vi "Assemble.vi"() -> ()   [LabVIEW 2010]
uses:
  <vilib>/Utility/VariantDataType/VariantType.lvlib
panel:
  out "Result: XML Footer":string
  out "Result: XML Header":string
  out "XML-String-out":string
  out "output array":variant[](array[variant])
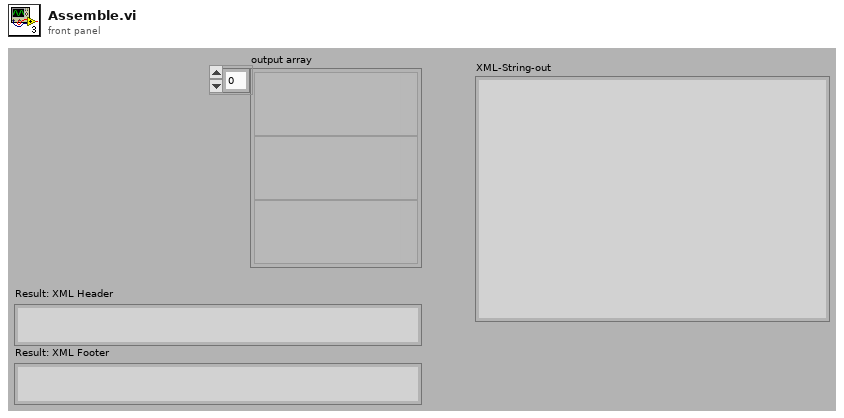
[diagram p1: front panel]
types:
  T1 = cluster{"parameter":string, "type info":string}[]
  T2 = typedef "VariantType.lvlib/Type.ctl" = enum8{"Invalid Type", "Void", "I8", "I16", "I32", "I64", "U8", "U16", "U32", "U64", "Single Float", "Double Float", "Extended Float", "Single Complex", "Double Complex", "Extended Complex", "Enum U8", "Enum U16", "Enum U32", "Enum U64", "Single Float With Unit", "Double Float With Unit", "Extended Float With Unit", "Single Complex with Unit", "Double Complex with Unit", "Extended Complex with Unit", "Boolean", "String", "Path", "Picture", "Tag", "Array", "Cluster", "Variant", "LV Variant", "Waveform", "Timestamp", "Digital Waveform", "Digital Data", "ExpressData", "Refnum", "External Data", "VI", "Poly VI", "LabVIEW Class Instance", "Fixed Point"}
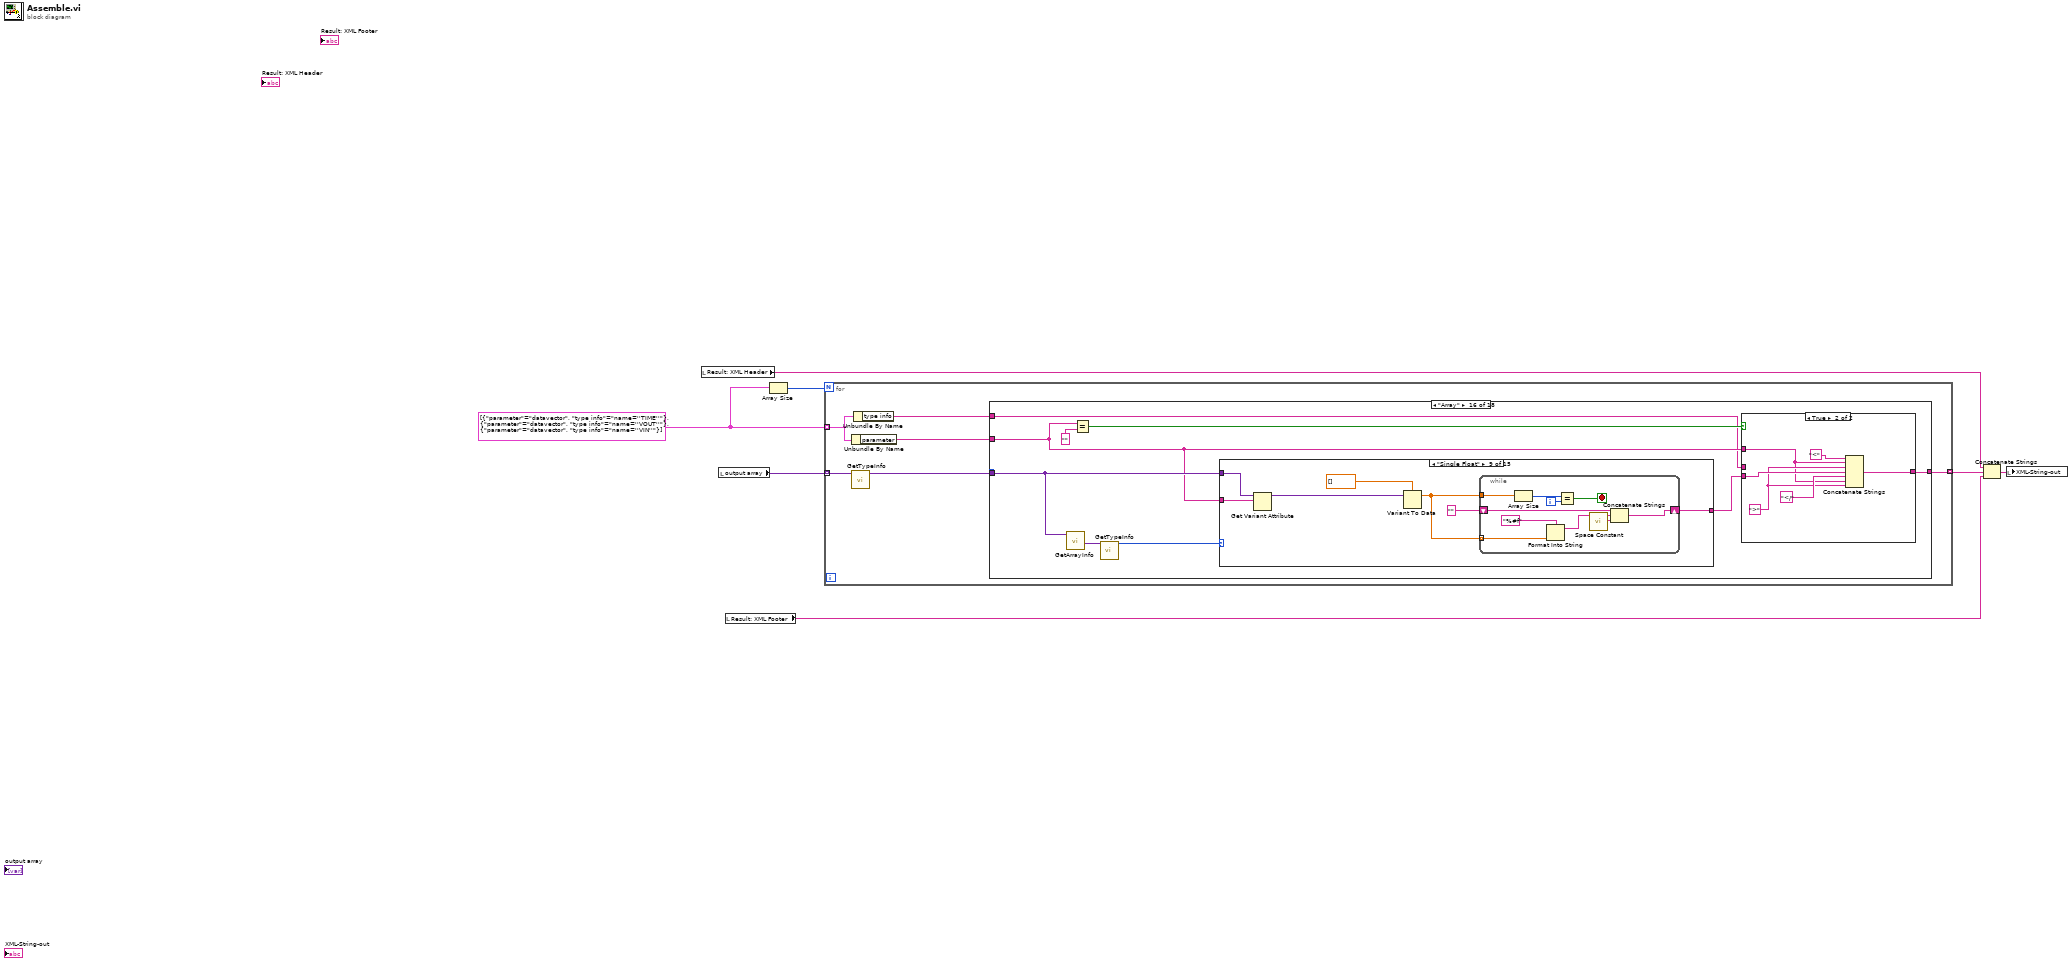
[diagram p0: block diagram]
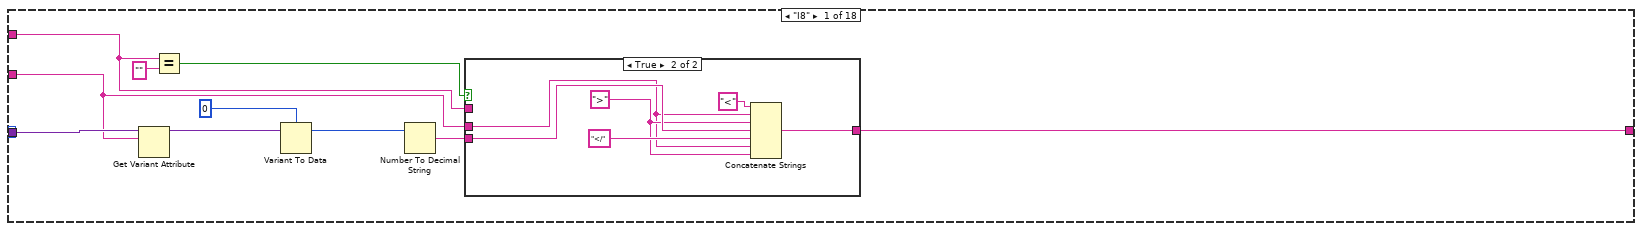
[diagram p2: hidden frame]
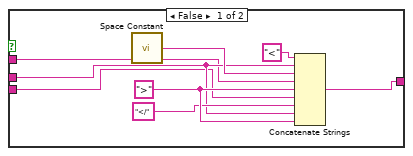
[diagram p3: hidden frame]
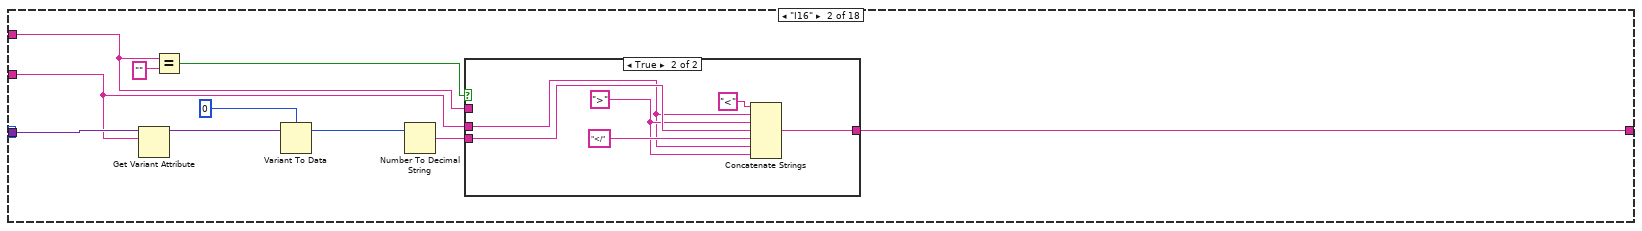
[diagram p4: hidden frame]
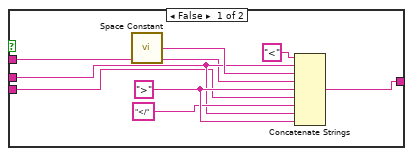
[diagram p5: hidden frame]
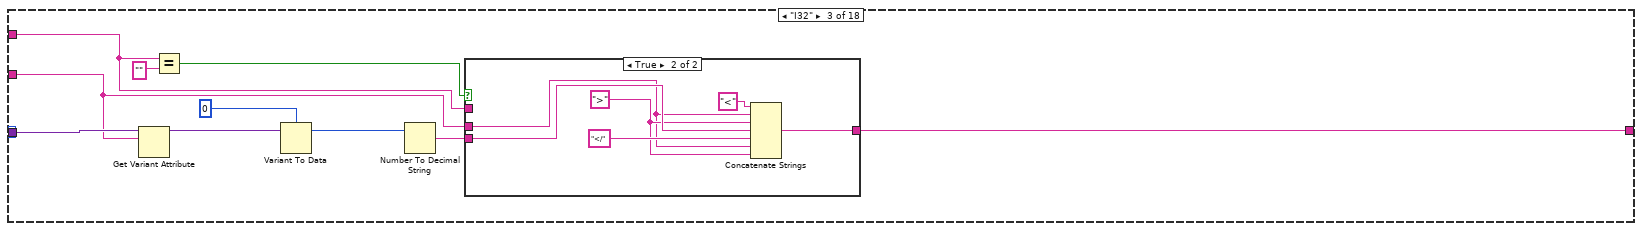
[diagram p6: hidden frame]
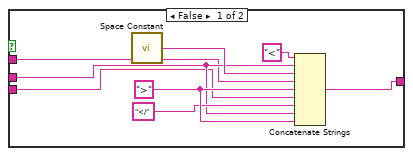
[diagram p7: hidden frame]
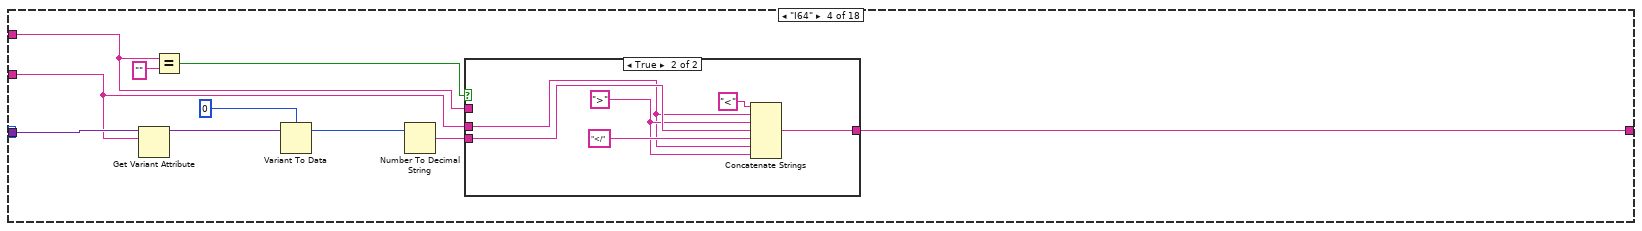
[diagram p8: hidden frame]
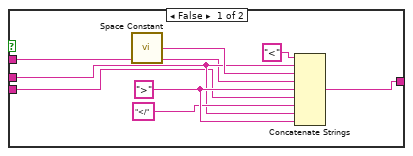
[diagram p9: hidden frame]
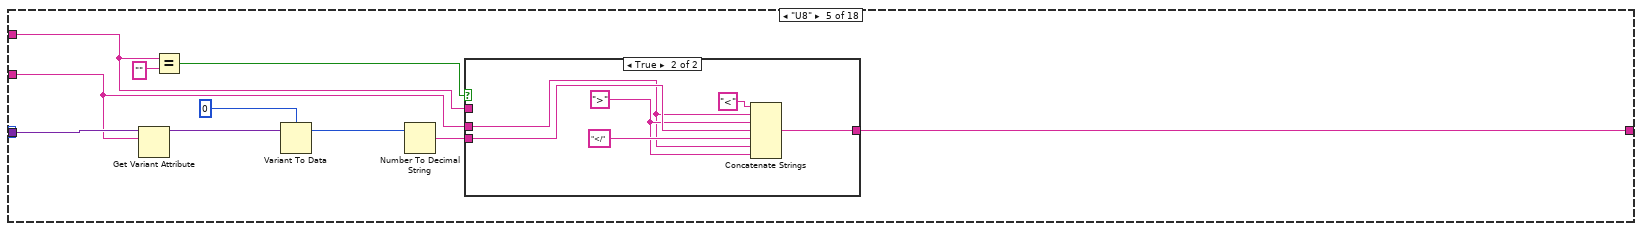
[diagram p10: hidden frame]
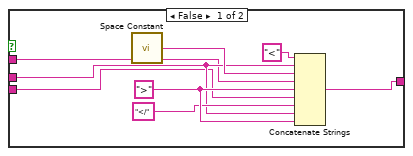
[diagram p11: hidden frame]
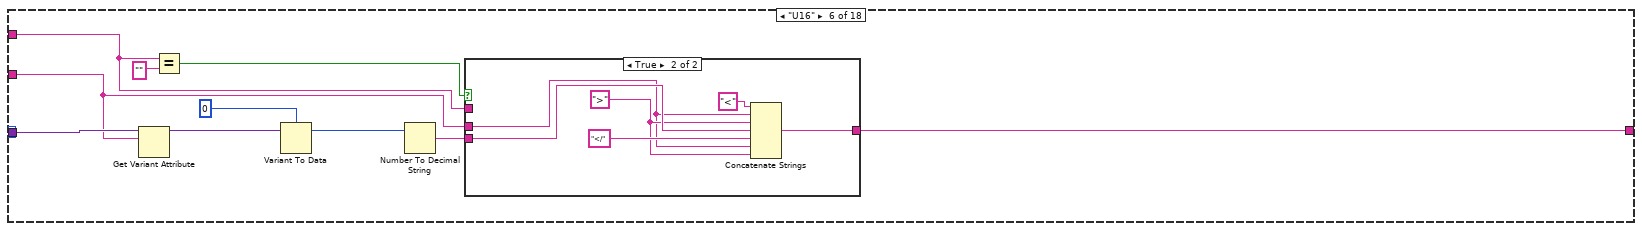
[diagram p12: hidden frame]
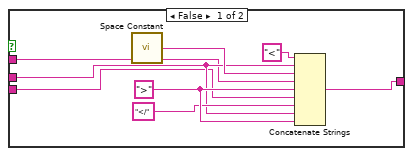
[diagram p13: hidden frame]
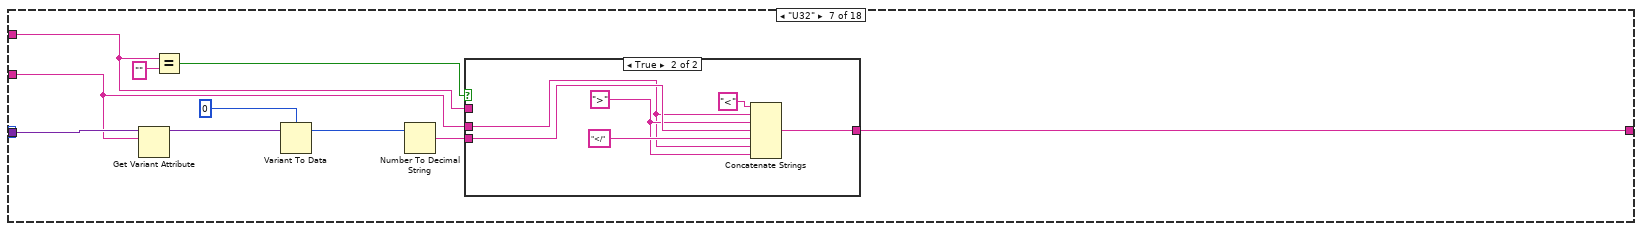
[diagram p14: hidden frame]
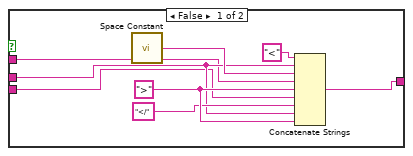
[diagram p15: hidden frame]
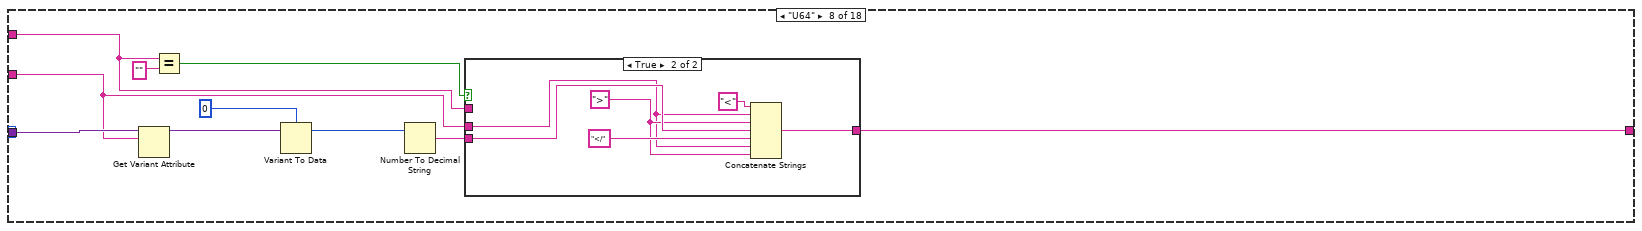
[diagram p16: hidden frame]
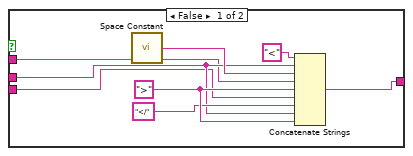
[diagram p17: hidden frame]
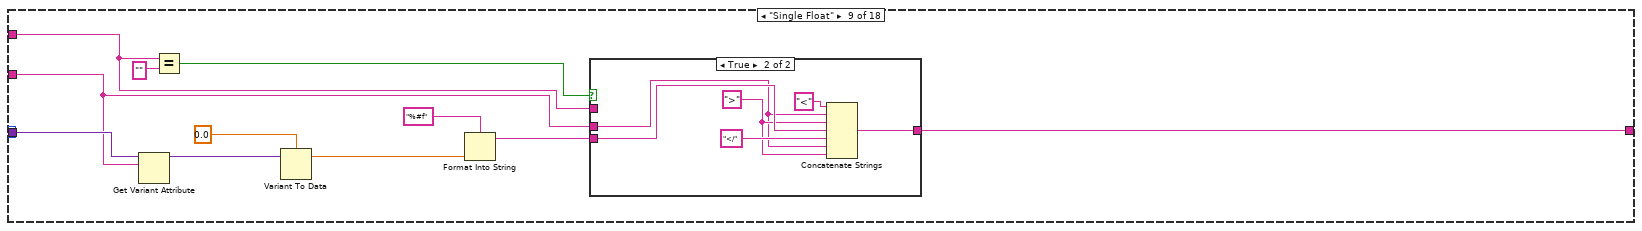
[diagram p18: hidden frame]
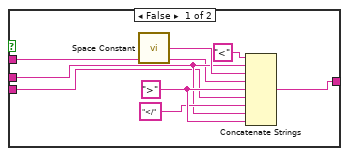
[diagram p19: hidden frame]
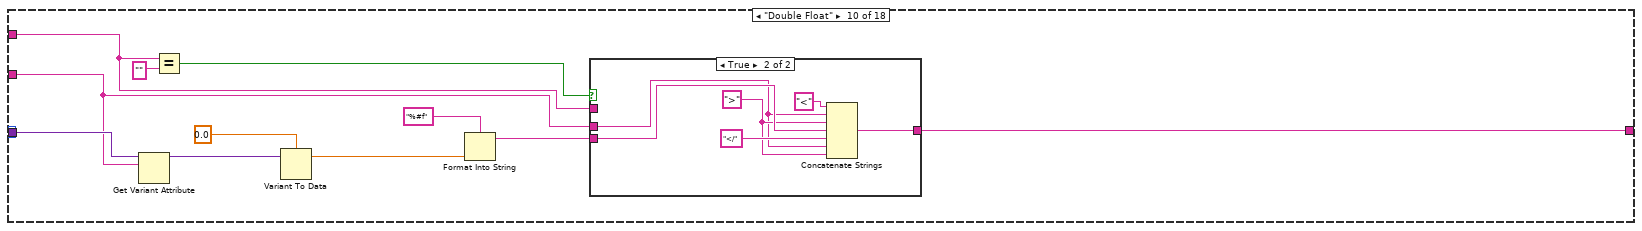
[diagram p20: hidden frame]
diagram:
  w1 = T1 [{"parameter"="datavector", "type info"="name=''TIME''"}, {"parameter"="datavector", "type info"="name=''VOUT''"}, {"parameter"="datavector", "type info"="name=''VIN''"}] ("Parameter out 2")
  n1 = local read "Result: XML Header"() -> (w3:string)
  n2 = local read "output array"() -> (w4:variant[])
  n3 = local read "Result: XML Footer"() -> (w2:string)
  n4 = Array Size(array=w1) -> (size(s)=w7:i32)
  n5 = for {
    N: w7 -> [_]
    tunnel: w4 -> [w11] mode=indexing
    tunnel: w1 -> [w9] mode=indexing
    tunnel: [w13] -> w5 mode=indexing
    n6 = Unbundle By Name(w9) -> ("parameter"=w12:string)
    n7 = call <vilib>:"GetTypeInfo.vi"("Variant"=w11) -> ("Type Enum"=w10:T2)  [unwired: 6 in, 4 out]
    n8 = Unbundle By Name(w9) -> ("type info"=w8:string)
    n9 = case shown="\"Array\"" w10 {
      tunnel: w12 -> [w15 w39 w64 w87 w112 w135 w159 w183 w207 w232 w257 w282 w306 w330 w354 w379 w647 w667]
      tunnel: [w14 w38 w62 w86 w111 w134 w158 w182 w206 w231 w256 w281 w305 w329 w353 w383 w643 w666] -> w13
      tunnel: w11 -> [w20 w44 w68 w92 w116 w140 w164 w188 w214 w239 w264 w287 w311 w335 w359 w384 w649 w675]
      tunnel: w8 -> [w17 w41 w65 w89 w110 w137 w161 w185 w209 w234 w259 w284 w308 w332 w356 w378 w645 w669]
      frame "I8" {
        n10 = Get Variant Attribute(Variant=w20, name=w15) -> (duplicate Variant=w21:variant)  [unwired: 2 in, 3 out]
        n11 = Equal?(x=w17, y="") -> (x = y?=w19:bool)
        n12 = Variant To Data(Variant=w21, type=i8 0) -> (data=w23:i8)  [unwired: 1 in, 1 out]
        n13 = Number To Decimal String(number=w23) -> (decimal integer string=w16:string)  [unwired: 1 in]
        n14 = case shown="True" w19 {
          tunnel: w15 -> [w27 w32]
          tunnel: w17 -> [w24 _]
          tunnel: w16 -> [w26 w35]
          tunnel: [w25 w36] -> w14
          frame False {
            w30 = ">" ("string")
            n15 = call <vilib>:"Space Constant.vi"() -> ("String"=w31:string)
            n16 = Concatenate Strings("<" ("string"), w27, w31, w24, w30, w26, "</" ("string"), w27, w30) -> (w25:string)
          }
          frame True {
            w33 = ">" ("string")
            n17 = Concatenate Strings("<" ("string"), w32, w33, w35, "</" ("string"), w32, w33) -> (w36:string)
          }
        }
      }
      frame "I16" {
        n18 = Get Variant Attribute(Variant=w44, name=w39) -> (duplicate Variant=w46:variant)  [unwired: 2 in, 3 out]
        n19 = Equal?(x=w41, y="") -> (x = y?=w43:bool)
        n20 = Variant To Data(Variant=w46, type=i16 0 ("I16")) -> (data=w47:i16)  [unwired: 1 in, 1 out]
        n21 = Number To Decimal String(number=w47) -> (decimal integer string=w40:string)  [unwired: 1 in]
        n22 = case shown="True" w43 {
          tunnel: w39 -> [w51 w56]
          tunnel: w41 -> [w48 _]
          tunnel: w40 -> [w50 w59]
          tunnel: [w49 w60] -> w38
          frame False {
            w54 = ">" ("string")
            n23 = call <vilib>:"Space Constant.vi"() -> ("String"=w55:string)
            n24 = Concatenate Strings("<" ("string"), w51, w55, w48, w54, w50, "</" ("string"), w51, w54) -> (w49:string)
          }
          frame True {
            w57 = ">" ("string")
            n25 = Concatenate Strings("<" ("string"), w56, w57, w59, "</" ("string"), w56, w57) -> (w60:string)
          }
        }
      }
      frame "I32" {
        n26 = Get Variant Attribute(Variant=w68, name=w64) -> (duplicate Variant=w69:variant)  [unwired: 2 in, 3 out]
        n27 = Equal?(x=w65, y="") -> (x = y?=w67:bool)
        n28 = Variant To Data(Variant=w69, type=i16 0 ("precision (6)")) -> (data=w71:i16)  [unwired: 1 in, 1 out]
        n29 = Number To Decimal String(number=w71) -> (decimal integer string=w63:string)  [unwired: 1 in]
        n30 = case shown="True" w67 {
          tunnel: w64 -> [w75 w80]
          tunnel: w65 -> [w72 _]
          tunnel: w63 -> [w74 w83]
          tunnel: [w73 w84] -> w62
          frame False {
            w78 = ">" ("string")
            n31 = call <vilib>:"Space Constant.vi"() -> ("String"=w79:string)
            n32 = Concatenate Strings("<" ("string"), w75, w79, w72, w78, w74, "</" ("string"), w75, w78) -> (w73:string)
          }
          frame True {
            w81 = ">" ("string")
            n33 = Concatenate Strings("<" ("string"), w80, w81, w83, "</" ("string"), w80, w81) -> (w84:string)
          }
        }
      }
      frame "I64" {
        n34 = Get Variant Attribute(Variant=w92, name=w87) -> (duplicate Variant=w93:variant)  [unwired: 2 in, 3 out]
        n35 = Equal?(x=w89, y="") -> (x = y?=w91:bool)
        n36 = Variant To Data(Variant=w93, type=i64 0) -> (data=w95:i64)  [unwired: 1 in, 1 out]
        n37 = Number To Decimal String(number=w95) -> (decimal integer string=w88:string)  [unwired: 1 in]
        n38 = case shown="True" w91 {
          tunnel: w87 -> [w99 w104]
          tunnel: w89 -> [w96 _]
          tunnel: w88 -> [w98 w107]
          tunnel: [w97 w108] -> w86
          frame False {
            w102 = ">" ("string")
            n39 = call <vilib>:"Space Constant.vi"() -> ("String"=w103:string)
            n40 = Concatenate Strings("<" ("string"), w99, w103, w96, w102, w98, "</" ("string"), w99, w102) -> (w97:string)
          }
          frame True {
            w105 = ">" ("string")
            n41 = Concatenate Strings("<" ("string"), w104, w105, w107, "</" ("string"), w104, w105) -> (w108:string)
          }
        }
      }
      frame "U8" {
        n42 = Get Variant Attribute(Variant=w116, name=w112) -> (duplicate Variant=w117:variant)  [unwired: 2 in, 3 out]
        n43 = Equal?(x=w110, y="") -> (x = y?=w115:bool)
        n44 = Variant To Data(Variant=w117, type=u8 0) -> (data=w119:u8)  [unwired: 1 in, 1 out]
        n45 = Number To Decimal String(number=w119) -> (decimal integer string=w113:string)  [unwired: 1 in]
        n46 = case shown="True" w115 {
          tunnel: w112 -> [w123 w128]
          tunnel: w110 -> [w120 _]
          tunnel: w113 -> [w122 w131]
          tunnel: [w121 w132] -> w111
          frame False {
            w126 = ">" ("string")
            n47 = call <vilib>:"Space Constant.vi"() -> ("String"=w127:string)
            n48 = Concatenate Strings("<" ("string"), w123, w127, w120, w126, w122, "</" ("string"), w123, w126) -> (w121:string)
          }
          frame True {
            w129 = ">" ("string")
            n49 = Concatenate Strings("<" ("string"), w128, w129, w131, "</" ("string"), w128, w129) -> (w132:string)
          }
        }
      }
      frame "U16" {
        n50 = Get Variant Attribute(Variant=w140, name=w135) -> (duplicate Variant=w141:variant)  [unwired: 2 in, 3 out]
        n51 = Equal?(x=w137, y="") -> (x = y?=w139:bool)
        n52 = Variant To Data(Variant=w141, type=u16 0) -> (data=w143:u16)  [unwired: 1 in, 1 out]
        n53 = Number To Decimal String(number=w143) -> (decimal integer string=w136:string)  [unwired: 1 in]
        n54 = case shown="True" w139 {
          tunnel: w135 -> [w147 w152]
          tunnel: w137 -> [w144 _]
          tunnel: w136 -> [w146 w155]
          tunnel: [w145 w156] -> w134
          frame False {
            w150 = ">" ("string")
            n55 = call <vilib>:"Space Constant.vi"() -> ("String"=w151:string)
            n56 = Concatenate Strings("<" ("string"), w147, w151, w144, w150, w146, "</" ("string"), w147, w150) -> (w145:string)
          }
          frame True {
            w153 = ">" ("string")
            n57 = Concatenate Strings("<" ("string"), w152, w153, w155, "</" ("string"), w152, w153) -> (w156:string)
          }
        }
      }
      frame "U32" {
        n58 = Get Variant Attribute(Variant=w164, name=w159) -> (duplicate Variant=w165:variant)  [unwired: 2 in, 3 out]
        n59 = Equal?(x=w161, y="") -> (x = y?=w163:bool)
        n60 = Variant To Data(Variant=w165, type=u32 0) -> (data=w167:u32)  [unwired: 1 in, 1 out]
        n61 = Number To Decimal String(number=w167) -> (decimal integer string=w160:string)  [unwired: 1 in]
        n62 = case shown="True" w163 {
          tunnel: w159 -> [w171 w176]
          tunnel: w161 -> [w168 _]
          tunnel: w160 -> [w170 w179]
          tunnel: [w169 w180] -> w158
          frame False {
            w174 = ">" ("string")
            n63 = call <vilib>:"Space Constant.vi"() -> ("String"=w175:string)
            n64 = Concatenate Strings("<" ("string"), w171, w175, w168, w174, w170, "</" ("string"), w171, w174) -> (w169:string)
          }
          frame True {
            w177 = ">" ("string")
            n65 = Concatenate Strings("<" ("string"), w176, w177, w179, "</" ("string"), w176, w177) -> (w180:string)
          }
        }
      }
      frame "U64" {
        n66 = Get Variant Attribute(Variant=w188, name=w183) -> (duplicate Variant=w189:variant)  [unwired: 2 in, 3 out]
        n67 = Equal?(x=w185, y="") -> (x = y?=w187:bool)
        n68 = Variant To Data(Variant=w189, type=u64 0) -> (data=w191:u64)  [unwired: 1 in, 1 out]
        n69 = Number To Decimal String(number=w191) -> (decimal integer string=w184:string)  [unwired: 1 in]
        n70 = case shown="True" w187 {
          tunnel: w183 -> [w195 w200]
          tunnel: w185 -> [w192 _]
          tunnel: w184 -> [w194 w203]
          tunnel: [w193 w204] -> w182
          frame False {
            w198 = ">" ("string")
            n71 = call <vilib>:"Space Constant.vi"() -> ("String"=w199:string)
            n72 = Concatenate Strings("<" ("string"), w195, w199, w192, w198, w194, "</" ("string"), w195, w198) -> (w193:string)
          }
          frame True {
            w201 = ">" ("string")
            n73 = Concatenate Strings("<" ("string"), w200, w201, w203, "</" ("string"), w200, w201) -> (w204:string)
          }
        }
      }
      frame "Single Float" {
        n74 = Get Variant Attribute(Variant=w214, name=w207) -> (duplicate Variant=w215:variant)  [unwired: 2 in, 3 out]
        n75 = Equal?(x=w209, y="") -> (x = y?=w211:bool)
        n76 = Variant To Data(Variant=w215, type=sgl 0.0) -> (data=w212:sgl)  [unwired: 1 in, 1 out]
        n77 = Format Into String(format string="%#f", w212) -> (resulting string=w208:string)  [unwired: 2 in, 1 out]
        n78 = case shown="True" w211 {
          tunnel: w207 -> [w220 w225]
          tunnel: w209 -> [w217 _]
          tunnel: w208 -> [w219 w228]
          tunnel: [w218 w229] -> w206
          frame False {
            w223 = ">" ("string")
            n79 = call <vilib>:"Space Constant.vi"() -> ("String"=w224:string)
            n80 = Concatenate Strings("<" ("string"), w220, w224, w217, w223, w219, "</" ("string"), w220, w223) -> (w218:string)
          }
          frame True {
            w226 = ">" ("string")
            n81 = Concatenate Strings("<" ("string"), w225, w226, w228, "</" ("string"), w225, w226) -> (w229:string)
          }
        }
      }
      frame "Double Float" {
        n82 = Get Variant Attribute(Variant=w239, name=w232) -> (duplicate Variant=w240:variant)  [unwired: 2 in, 3 out]
        n83 = Equal?(x=w234, y="") -> (x = y?=w236:bool)
        n84 = Variant To Data(Variant=w240, type=0.0) -> (data=w237:dbl)  [unwired: 1 in, 1 out]
        n85 = Format Into String(format string="%#f", w237) -> (resulting string=w233:string)  [unwired: 2 in, 1 out]
        n86 = case shown="True" w236 {
          tunnel: w232 -> [w245 w250]
          tunnel: w234 -> [w242 _]
          tunnel: w233 -> [w244 w253]
          tunnel: [w243 w254] -> w231
          frame False {
            w248 = ">" ("string")
            n87 = call <vilib>:"Space Constant.vi"() -> ("String"=w249:string)
            n88 = Concatenate Strings("<" ("string"), w245, w249, w242, w248, w244, "</" ("string"), w245, w248) -> (w243:string)
          }
          frame True {
            w251 = ">" ("string")
            n89 = Concatenate Strings("<" ("string"), w250, w251, w253, "</" ("string"), w250, w251) -> (w254:string)
          }
        }
      }
      frame "Extended Float" {
        n90 = Get Variant Attribute(Variant=w264, name=w257) -> (duplicate Variant=w265:variant)  [unwired: 2 in, 3 out]
        n91 = Equal?(x=w259, y="") -> (x = y?=w261:bool)
        n92 = Variant To Data(Variant=w265, type=ext 0.0) -> (data=w262:ext)  [unwired: 1 in, 1 out]
        n93 = Format Into String(format string="%#f", w262) -> (resulting string=w258:string)  [unwired: 2 in, 1 out]
        n94 = case shown="True" w261 {
          tunnel: w257 -> [w270 w275]
          tunnel: w259 -> [w267 _]
          tunnel: w258 -> [w269 w278]
          tunnel: [w268 w279] -> w256
          frame False {
            w273 = ">" ("string")
            n95 = call <vilib>:"Space Constant.vi"() -> ("String"=w274:string)
            n96 = Concatenate Strings("<" ("string"), w270, w274, w267, w273, w269, "</" ("string"), w270, w273) -> (w268:string)
          }
          frame True {
            w276 = ">" ("string")
            n97 = Concatenate Strings("<" ("string"), w275, w276, w278, "</" ("string"), w275, w276) -> (w279:string)
          }
        }
      }
      frame "Single Complex" {
        n98 = Get Variant Attribute(Variant=w287, name=w282) -> (duplicate Variant=w288:variant)  [unwired: 2 in, 3 out]
        n99 = Equal?(x=w284, y="") -> (x = y?=w286:bool)
        n100 = Variant To Data(Variant=w288, type=csg 0.0+0.0i ("number 3")) -> (data=w290:csg)  [unwired: 1 in, 1 out]
        n101 = Format Value(value (0)=w290) -> (output string=w283:string)  [unwired: 2 in]
        n102 = case shown="True" w286 {
          tunnel: w282 -> [w294 w299]
          tunnel: w284 -> [w291 _]
          tunnel: w283 -> [w293 w302]
          tunnel: [w292 w303] -> w281
          frame False {
            w297 = ">" ("string")
            n103 = call <vilib>:"Space Constant.vi"() -> ("String"=w298:string)
            n104 = Concatenate Strings("<" ("string"), w294, w298, w291, w297, w293, "</" ("string"), w294, w297) -> (w292:string)
          }
          frame True {
            w300 = ">" ("string")
            n105 = Concatenate Strings("<" ("string"), w299, w300, w302, "</" ("string"), w299, w300) -> (w303:string)
          }
        }
      }
      frame "Double Complex" {
        n106 = Get Variant Attribute(Variant=w311, name=w306) -> (duplicate Variant=w312:variant)  [unwired: 2 in, 3 out]
        n107 = Equal?(x=w308, y="") -> (x = y?=w310:bool)
        n108 = Variant To Data(Variant=w312, type=cdb 0.0+0.0i ("number 3")) -> (data=w314:cdb)  [unwired: 1 in, 1 out]
        n109 = Format Value(value (0)=w314) -> (output string=w307:string)  [unwired: 2 in]
        n110 = case shown="True" w310 {
          tunnel: w306 -> [w318 w323]
          tunnel: w308 -> [w315 _]
          tunnel: w307 -> [w317 w326]
          tunnel: [w316 w327] -> w305
          frame False {
            w321 = ">" ("string")
            n111 = call <vilib>:"Space Constant.vi"() -> ("String"=w322:string)
            n112 = Concatenate Strings("<" ("string"), w318, w322, w315, w321, w317, "</" ("string"), w318, w321) -> (w316:string)
          }
          frame True {
            w324 = ">" ("string")
            n113 = Concatenate Strings("<" ("string"), w323, w324, w326, "</" ("string"), w323, w324) -> (w327:string)
          }
        }
      }
      frame "Extended Complex" {
        n114 = Get Variant Attribute(Variant=w335, name=w330) -> (duplicate Variant=w336:variant)  [unwired: 2 in, 3 out]
        n115 = Equal?(x=w332, y="") -> (x = y?=w334:bool)
        n116 = Variant To Data(Variant=w336, type=cxt 0.0+0.0i ("number 3")) -> (data=w337:cxt)  [unwired: 1 in, 1 out]
        n117 = Format Value(value (0)=w337) -> (output string=w331:string)  [unwired: 2 in]
        n118 = case shown="True" w334 {
          tunnel: w330 -> [w342 w347]
          tunnel: w332 -> [w339 _]
          tunnel: w331 -> [w341 w350]
          tunnel: [w340 w351] -> w329
          frame False {
            w345 = ">" ("string")
            n119 = call <vilib>:"Space Constant.vi"() -> ("String"=w346:string)
            n120 = Concatenate Strings("<" ("string"), w342, w346, w339, w345, w341, "</" ("string"), w342, w345) -> (w340:string)
          }
          frame True {
            w348 = ">" ("string")
            n121 = Concatenate Strings("<" ("string"), w347, w348, w350, "</" ("string"), w347, w348) -> (w351:string)
          }
        }
      }
      frame "Boolean" {
        n122 = Get Variant Attribute(Variant=w359, name=w354) -> (duplicate Variant=w360:variant)  [unwired: 2 in, 3 out]
        n123 = Equal?(x=w356, y="") -> (x = y?=w358:bool)
        n124 = Variant To Data(Variant=w360, type=TRUE) -> (data=w363:bool)  [unwired: 1 in, 1 out]
        n125 = Boolean To (0,1)(Boolean=w363) -> (0, 1=w361:i16)
        n126 = Number To Decimal String(number=w361) -> (decimal integer string=w355:string)  [unwired: 1 in]
        n127 = case shown="True" w358 {
          tunnel: w354 -> [w367 w372]
          tunnel: w356 -> [w364 _]
          tunnel: w355 -> [w366 w375]
          tunnel: [w365 w376] -> w353
          frame False {
            w370 = ">" ("string")
            n128 = call <vilib>:"Space Constant.vi"() -> ("String"=w371:string)
            n129 = Concatenate Strings("<" ("string"), w367, w371, w364, w370, w366, "</" ("string"), w367, w370) -> (w365:string)
          }
          frame True {
            w373 = ">" ("string")
            n130 = Concatenate Strings("<" ("string"), w372, w373, w375, "</" ("string"), w372, w373) -> (w376:string)
          }
        }
      }
      frame "Array" {
        n131 = call <vilib>:"GetArrayInfo.vi"("Variant"=w384) -> ("ArrayElement"=w386:variant)  [unwired: 7 in, 3 out]
        n132 = Equal?(x=w379, y="") -> (x = y?=w382:bool)
        n133 = call <vilib>:"GetTypeInfo.vi"("Variant"=w386) -> ("Type Enum"=w385:T2)  [unwired: 6 in, 4 out]
        n134 = case shown="\"Single Float\"" w385 {
          tunnel: w384 -> [w407 w422 w435 w451 w466 w483 w498 w515 w530 w547 w565 w582 w598 w614 w632]
          tunnel: [w402 w420 w433 w449 w467 w481 w499 w513 w532 w548 w563 w580 w596 w612 w628] -> w380
          tunnel: w379 -> [w401 w417 w434 w450 w465 w482 w497 w514 w529 w546 w564 w581 w597 w613 w631]
          frame "I8" {
            n135 = Get Variant Attribute(Variant=w407, name=w401) -> (duplicate Variant=w406:variant)  [unwired: 2 in, 3 out]
            n136 = Variant To Data(Variant=w406, type=u8[] [] ("Array")) -> (data=w404:u8[])  [unwired: 1 in, 1 out]
            n137 = while {
              tunnel: w404 -> [w416] mode=indexing
              tunnel: w404 -> [w415]
              shift-right: [w408] -> w402
              shift-left: "" -> [w409]
              i -> [w413]
              stop <- w412 stop-if-true
              n138 = Array Size(array=w415) -> (size(s)=w414:i32)
              n139 = Number To Decimal String(number=w416) -> (decimal integer string=w411:string)  [unwired: 1 in]
              n140 = call <vilib>:"Space Constant.vi"() -> ("String"=w410:string)
              n141 = Equal?(x=w414, y=w413) -> (x = y?=w412:bool)
              n142 = Concatenate Strings(w409, w411, w410) -> (w408:string)
            }
          }
          frame "I16" {
            n143 = Get Variant Attribute(Variant=w422, name=w417) -> (duplicate Variant=w419:variant)  [unwired: 2 in, 3 out]
            n144 = Variant To Data(Variant=w419, type=i16[] [] ("Array")) -> (data=w418:i16[])  [unwired: 1 in, 1 out]
            n145 = while {
              tunnel: w418 -> [w432] mode=indexing
              shift-right: [w425] -> w420
              shift-left: "" -> [w426]
              tunnel: w418 -> [w424]
              i -> [w430]
              stop <- w429 stop-if-true
              n146 = Array Size(array=w424) -> (size(s)=w431:i32)
              n147 = Number To Decimal String(number=w432) -> (decimal integer string=w428:string)  [unwired: 1 in]
              n148 = call <vilib>:"Space Constant.vi"() -> ("String"=w427:string)
              n149 = Equal?(x=w431, y=w430) -> (x = y?=w429:bool)
              n150 = Concatenate Strings(w426, w428, w427) -> (w425:string)
            }
          }
          frame "I32" {
            n151 = Get Variant Attribute(Variant=w435, name=w434) -> (duplicate Variant=w437:variant)  [unwired: 2 in, 3 out]
            n152 = Variant To Data(Variant=w437, type=i16[] [] ("Array")) -> (data=w436:i16[])  [unwired: 1 in, 1 out]
            n153 = while {
              tunnel: w436 -> [w448] mode=indexing
              shift-right: [w441] -> w433
              shift-left: "" -> [w442]
              tunnel: w436 -> [w440]
              i -> [w446]
              stop <- w445 stop-if-true
              n154 = Array Size(array=w440) -> (size(s)=w447:i32)
              n155 = Number To Decimal String(number=w448) -> (decimal integer string=w444:string)  [unwired: 1 in]
              n156 = call <vilib>:"Space Constant.vi"() -> ("String"=w443:string)
              n157 = Equal?(x=w447, y=w446) -> (x = y?=w445:bool)
              n158 = Concatenate Strings(w442, w444, w443) -> (w441:string)
            }
          }
          frame "I64" {
            n159 = Get Variant Attribute(Variant=w451, name=w450) -> (duplicate Variant=w453:variant)  [unwired: 2 in, 3 out]
            n160 = Variant To Data(Variant=w453, type=i64[] [] ("Array")) -> (data=w452:i64[])  [unwired: 1 in, 1 out]
            n161 = while {
              tunnel: w452 -> [w464] mode=indexing
              shift-right: [w457] -> w449
              shift-left: "" -> [w458]
              tunnel: w452 -> [w456]
              i -> [w462]
              stop <- w461 stop-if-true
              n162 = Array Size(array=w456) -> (size(s)=w463:i32)
              n163 = Number To Decimal String(number=w464) -> (decimal integer string=w460:string)  [unwired: 1 in]
              n164 = call <vilib>:"Space Constant.vi"() -> ("String"=w459:string)
              n165 = Equal?(x=w463, y=w462) -> (x = y?=w461:bool)
              n166 = Concatenate Strings(w458, w460, w459) -> (w457:string)
            }
          }
          frame "U8" {
            n167 = Get Variant Attribute(Variant=w466, name=w465) -> (duplicate Variant=w469:variant)  [unwired: 2 in, 3 out]
            n168 = Variant To Data(Variant=w469, type=u8[] [] ("Array")) -> (data=w468:u8[])  [unwired: 1 in, 1 out]
            n169 = while {
              tunnel: w468 -> [w480] mode=indexing
              shift-right: [w473] -> w467
              shift-left: "" -> [w474]
              tunnel: w468 -> [w472]
              i -> [w478]
              stop <- w477 stop-if-true
              n170 = Array Size(array=w472) -> (size(s)=w479:i32)
              n171 = Number To Decimal String(number=w480) -> (decimal integer string=w476:string)  [unwired: 1 in]
              n172 = call <vilib>:"Space Constant.vi"() -> ("String"=w475:string)
              n173 = Equal?(x=w479, y=w478) -> (x = y?=w477:bool)
              n174 = Concatenate Strings(w474, w476, w475) -> (w473:string)
            }
          }
          frame "U16" {
            n175 = Get Variant Attribute(Variant=w483, name=w482) -> (duplicate Variant=w485:variant)  [unwired: 2 in, 3 out]
            n176 = Variant To Data(Variant=w485, type=u16[] [] ("Array")) -> (data=w484:u16[])  [unwired: 1 in, 1 out]
            n177 = while {
              tunnel: w484 -> [w496] mode=indexing
              shift-right: [w489] -> w481
              shift-left: "" -> [w490]
              tunnel: w484 -> [w488]
              i -> [w494]
              stop <- w493 stop-if-true
              n178 = Array Size(array=w488) -> (size(s)=w495:i32)
              n179 = Number To Decimal String(number=w496) -> (decimal integer string=w492:string)  [unwired: 1 in]
              n180 = call <vilib>:"Space Constant.vi"() -> ("String"=w491:string)
              n181 = Equal?(x=w495, y=w494) -> (x = y?=w493:bool)
              n182 = Concatenate Strings(w490, w492, w491) -> (w489:string)
            }
          }
          frame "U32" {
            n183 = Get Variant Attribute(Variant=w498, name=w497) -> (duplicate Variant=w501:variant)  [unwired: 2 in, 3 out]
            n184 = Variant To Data(Variant=w501, type=u32[] [] ("Array")) -> (data=w500:u32[])  [unwired: 1 in, 1 out]
            n185 = while {
              tunnel: w500 -> [w512] mode=indexing
              shift-right: [w505] -> w499
              shift-left: "" -> [w506]
              tunnel: w500 -> [w504]
              i -> [w510]
              stop <- w509 stop-if-true
              n186 = Array Size(array=w504) -> (size(s)=w511:i32)
              n187 = Number To Decimal String(number=w512) -> (decimal integer string=w508:string)  [unwired: 1 in]
              n188 = call <vilib>:"Space Constant.vi"() -> ("String"=w507:string)
              n189 = Equal?(x=w511, y=w510) -> (x = y?=w509:bool)
              n190 = Concatenate Strings(w506, w508, w507) -> (w505:string)
            }
          }
          frame "U64" {
            n191 = Get Variant Attribute(Variant=w515, name=w514) -> (duplicate Variant=w517:variant)  [unwired: 2 in, 3 out]
            n192 = Variant To Data(Variant=w517, type=u64[] [] ("Array")) -> (data=w516:u64[])  [unwired: 1 in, 1 out]
            n193 = while {
              tunnel: w516 -> [w528] mode=indexing
              shift-right: [w521] -> w513
              shift-left: "" -> [w522]
              tunnel: w516 -> [w520]
              i -> [w526]
              stop <- w525 stop-if-true
              n194 = Array Size(array=w520) -> (size(s)=w527:i32)
              n195 = Number To Decimal String(number=w528) -> (decimal integer string=w524:string)  [unwired: 1 in]
              n196 = call <vilib>:"Space Constant.vi"() -> ("String"=w523:string)
              n197 = Equal?(x=w527, y=w526) -> (x = y?=w525:bool)
              n198 = Concatenate Strings(w522, w524, w523) -> (w521:string)
            }
          }
          frame "Single Float" {
            n199 = Get Variant Attribute(Variant=w530, name=w529) -> (duplicate Variant=w533:variant)  [unwired: 2 in, 3 out]
            n200 = Variant To Data(Variant=w533, type=sgl[] [] ("Array")) -> (data=w531:sgl[])  [unwired: 1 in, 1 out]
            n201 = while {
              tunnel: w531 -> [w537] mode=indexing
              shift-right: [w540] -> w532
              shift-left: "" -> [w541]
              tunnel: w531 -> [w539]
              i -> [w544]
              stop <- w543 stop-if-true
              n202 = Array Size(array=w539) -> (size(s)=w545:i32)
              n203 = Format Into String(format string="%#f", w537) -> (resulting string=w536:string)  [unwired: 2 in, 1 out]
              n204 = Equal?(x=w545, y=w544) -> (x = y?=w543:bool)
              n205 = call <vilib>:"Space Constant.vi"() -> ("String"=w542:string)
              n206 = Concatenate Strings(w541, w536, w542) -> (w540:string)
            }
          }
          frame "Double Float" {
            n207 = Get Variant Attribute(Variant=w547, name=w546) -> (duplicate Variant=w550:variant)  [unwired: 2 in, 3 out]
            n208 = Variant To Data(Variant=w550, type=dbl[] [] ("Array")) -> (data=w549:dbl[])  [unwired: 1 in, 1 out]
            n209 = while {
              tunnel: w549 -> [w554] mode=indexing
              shift-right: [w557] -> w548
              shift-left: "" -> [w558]
              tunnel: w549 -> [w556]
              i -> [w561]
              stop <- w560 stop-if-true
              n210 = Array Size(array=w556) -> (size(s)=w562:i32)
              n211 = Format Into String(format string="%f", w554) -> (resulting string=w553:string)  [unwired: 2 in, 1 out]
              n212 = Equal?(x=w562, y=w561) -> (x = y?=w560:bool)
              n213 = call <vilib>:"Space Constant.vi"() -> ("String"=w559:string)
              n214 = Concatenate Strings(w558, w553, w559) -> (w557:string)
            }
          }
          frame "Extended Float" {
            n215 = Get Variant Attribute(Variant=w565, name=w564) -> (duplicate Variant=w567:variant)  [unwired: 2 in, 3 out]
            n216 = Variant To Data(Variant=w567, type=ext[] [] ("Array")) -> (data=w566:ext[])  [unwired: 1 in, 1 out]
            n217 = while {
              tunnel: w566 -> [w571] mode=indexing
              shift-right: [w574] -> w563
              shift-left: "" -> [w575]
              tunnel: w566 -> [w573]
              i -> [w578]
              stop <- w577 stop-if-true
              n218 = Array Size(array=w573) -> (size(s)=w579:i32)
              n219 = Format Into String(format string="%#f", w571) -> (resulting string=w570:string)  [unwired: 2 in, 1 out]
              n220 = Equal?(x=w579, y=w578) -> (x = y?=w577:bool)
              n221 = call <vilib>:"Space Constant.vi"() -> ("String"=w576:string)
              n222 = Concatenate Strings(w575, w570, w576) -> (w574:string)
            }
          }
          frame "Single Complex" {
            n223 = Get Variant Attribute(Variant=w582, name=w581) -> (duplicate Variant=w584:variant)  [unwired: 2 in, 3 out]
            n224 = Variant To Data(Variant=w584, type=csg[] [] ("Array")) -> (data=w583:csg[])  [unwired: 1 in, 1 out]
            n225 = while {
              tunnel: w583 -> [w588] mode=indexing
              shift-right: [w590] -> w580
              shift-left: "" -> [w591]
              tunnel: w583 -> [w589]
              i -> [w594]
              stop <- w593 stop-if-true
              n226 = Array Size(array=w589) -> (size(s)=w595:i32)
              n227 = Format Value(value (0)=w588) -> (output string=w587:string)  [unwired: 2 in]
              n228 = call <vilib>:"Space Constant.vi"() -> ("String"=w592:string)
              n229 = Equal?(x=w595, y=w594) -> (x = y?=w593:bool)
              n230 = Concatenate Strings(w591, w587, w592) -> (w590:string)
            }
          }
          frame "Double Complex" {
            n231 = Get Variant Attribute(Variant=w598, name=w597) -> (duplicate Variant=w600:variant)  [unwired: 2 in, 3 out]
            n232 = Variant To Data(Variant=w600, type=cdb[] [] ("Array")) -> (data=w599:cdb[])  [unwired: 1 in, 1 out]
            n233 = while {
              tunnel: w599 -> [w604] mode=indexing
              shift-right: [w606] -> w596
              shift-left: "" -> [w607]
              tunnel: w599 -> [w605]
              i -> [w610]
              stop <- w609 stop-if-true
              n234 = Array Size(array=w605) -> (size(s)=w611:i32)
              n235 = Format Value(value (0)=w604) -> (output string=w603:string)  [unwired: 2 in]
              n236 = call <vilib>:"Space Constant.vi"() -> ("String"=w608:string)
              n237 = Equal?(x=w611, y=w610) -> (x = y?=w609:bool)
              n238 = Concatenate Strings(w607, w603, w608) -> (w606:string)
            }
          }
          frame "Extended Complex" {
            n239 = Get Variant Attribute(Variant=w614, name=w613) -> (duplicate Variant=w616:variant)  [unwired: 2 in, 3 out]
            n240 = Variant To Data(Variant=w616, type=cxt[] [] ("Array")) -> (data=w615:cxt[])  [unwired: 1 in, 1 out]
            n241 = while {
              tunnel: w615 -> [w620] mode=indexing
              shift-right: [w622] -> w612
              shift-left: "" -> [w623]
              tunnel: w615 -> [w621]
              i -> [w626]
              stop <- w625 stop-if-true
              n242 = Array Size(array=w621) -> (size(s)=w627:i32)
              n243 = Format Value(value (0)=w620) -> (output string=w619:string)  [unwired: 2 in]
              n244 = call <vilib>:"Space Constant.vi"() -> ("String"=w624:string)
              n245 = Equal?(x=w627, y=w626) -> (x = y?=w625:bool)
              n246 = Concatenate Strings(w623, w619, w624) -> (w622:string)
            }
          }
          frame "String", Default {
            n247 = Get Variant Attribute(Variant=w632, name=w631) -> (duplicate Variant=w633:variant)  [unwired: 2 in, 3 out]
            n248 = Variant To Data(Variant=w633, type=string[] [] ("Array")) -> (data=w629:string[])  [unwired: 1 in, 1 out]
            n249 = while {
              tunnel: w629 -> [w635] mode=indexing
              shift-right: [w637] -> w628
              shift-left: "" -> [w638]
              tunnel: w629 -> [w636]
              i -> [w641]
              stop <- w640 stop-if-true
              n250 = call <vilib>:"Space Constant.vi"() -> ("String"=w639:string)
              n251 = Array Size(array=w636) -> (size(s)=w642:i32)
              n252 = Concatenate Strings(w638, w635, w639) -> (w637:string)
              n253 = Equal?(x=w642, y=w641) -> (x = y?=w640:bool)
            }
          }
        }
        n254 = case shown="True" w382 {
          tunnel: w379 -> [w390 w395]
          tunnel: w378 -> [w387 _]
          tunnel: w380 -> [w389 w398]
          tunnel: [w388 w399] -> w383
          frame False {
            w393 = ">" ("string")
            n255 = call <vilib>:"Space Constant.vi"() -> ("String"=w394:string)
            n256 = Concatenate Strings("<" ("string"), w390, w394, w387, w393, w389, "</" ("string"), w390, w393) -> (w388:string)
          }
          frame True {
            w396 = ">" ("string")
            n257 = Concatenate Strings("<" ("string"), w395, w396, w398, "</" ("string"), w395, w396) -> (w399:string)
          }
        }
      }
      frame "String", Default {
        n258 = Get Variant Attribute(Variant=w649, name=w647) -> (duplicate Variant=w650:variant)  [unwired: 2 in, 3 out]
        n259 = Equal?(x=w645, y="") -> (x = y?=w646:bool)
        n260 = Variant To Data(Variant=w650, type="") -> (data=w648:string)  [unwired: 1 in, 1 out]
        n261 = case shown="True" w646 {
          tunnel: w647 -> [w655 w660]
          tunnel: w645 -> [w652 _]
          tunnel: w648 -> [w654 w663]
          tunnel: [w653 w664] -> w643
          frame False {
            w658 = ">" ("string")
            n262 = call <vilib>:"Space Constant.vi"() -> ("String"=w659:string)
            n263 = Concatenate Strings("<" ("string"), w655, w659, w652, w658, w654, "</" ("string"), w655, w658) -> (w653:string)
          }
          frame True {
            w661 = ">" ("string")
            n264 = Concatenate Strings("<" ("string"), w660, w661, w663, "</" ("string"), w660, w661) -> (w664:string)
          }
        }
      }
      frame "Fixed Point" {
        n265 = Get Variant Attribute(Variant=w675, name=w667) -> (duplicate Variant=w676:variant)  [unwired: 2 in, 3 out]
        n266 = Equal?(x=w669, y="") -> (x = y?=w671:bool)
        n267 = Variant To Data(Variant=w676, type=fxp<+,1,1> 0.0) -> (data=w673:fxp<+,1,1>)  [unwired: 1 in, 1 out]
        n268 = Format Into String(format string="%#f", w673) -> (resulting string=w668:string)  [unwired: 2 in, 1 out]
        n269 = case shown="True" w671 {
          tunnel: w667 -> [w680 w685]
          tunnel: w669 -> [w677 _]
          tunnel: w668 -> [w679 w688]
          tunnel: [w678 w689] -> w666
          frame False {
            w683 = ">" ("string")
            n270 = call <vilib>:"Space Constant.vi"() -> ("String"=w684:string)
            n271 = Concatenate Strings("<" ("string"), w680, w684, w677, w683, w679, "</" ("string"), w680, w683) -> (w678:string)
          }
          frame True {
            w686 = ">" ("string")
            n272 = Concatenate Strings("<" ("string"), w685, w686, w688, "</" ("string"), w685, w686) -> (w689:string)
          }
        }
      }
    }
  }
  n273 = Concatenate Strings(w3, w5, w2) -> (w6:string)
  n274 = local write "XML-String-out"(w6) -> ()
